vi "Snap to top.vi"(8 "centered? (F)":bool, 9 "Fixed Rect":T1, 11 "Rect":T1) -> (1 "TopLeft point":cluster{"x":i32, "y":i32}, 3 "Snapped to top":T1)   [LabVIEW 2012]
doc: "This VI calculates the position of a snapped-to-top rectangle from the positions of a large rectangle and a smaller one that will be positioned inside."
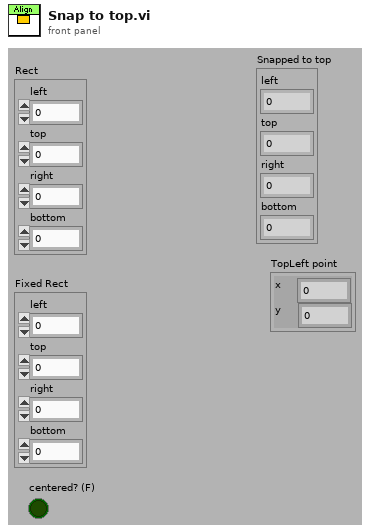
[diagram p1: front panel]
types:
  T1 = cluster{"left":i16, "top":i16, "right":i16, "bottom":i16}
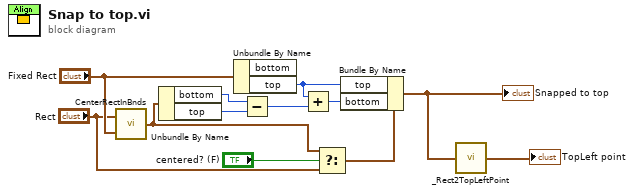
[diagram p0: block diagram]
diagram:
  n1 = call <vilib>:"CenterRectInBnds.vi"("bounds"="Fixed Rect", "rect"="Rect") -> ("centered rect"=w5:T1)
  n2 = Unbundle By Name(w5) -> ("bottom"=w12:i16, "top"=w11:i16)
  n3 = Unbundle By Name("Fixed Rect") -> ("top"=w8:i16)  [unwired: 1 out]
  n4 = Subtract(x=w12, y=w11) -> (x-y=w10:i16)
  n5 = Add(x=w8, y=w10) -> (x+y=w9:i16)
  n6 = Select(t=w5, s="centered? (F)", f="Rect") -> (s? t:f=w4:T1)
  n7 = Bundle By Name(cluster=w4, "top"=w8, "bottom"=w9) -> (w7:T1)
  "Snapped to top" <- w7
  n8 = call "_Rect2TopLeftPoint.vi"("bounds"=w7) -> ("TopLeft point"=→"TopLeft point":cluster{"x":i32, "y":i32})  [unwired: 4 out]
